vi "ASCII字符串转十六进制数组.vi"(11 "字符":string) -> (3 "数组":u8[](array[numeric]))   [LabVIEW 2015]
panel:
  out "长度":i32
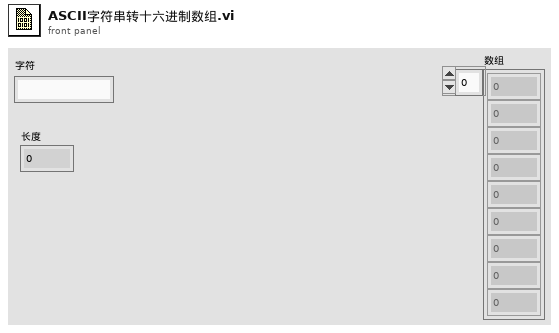
[diagram p1: front panel]
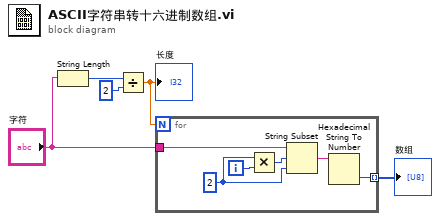
[diagram p0: block diagram]
diagram:
  n1 = String Length(string="字符") -> (length=w3:i32)
  n2 = Divide(x=w3, y=2) -> (x/y=w1:dbl)
  "长度" <- w1
  n3 = for {
    N: w1 -> [_]
    tunnel: "字符" -> [w8]
    tunnel: [w6] -> w4 mode=indexing
    i -> [w11]
    w10 = 2 ("长度（剩余）")
    n4 = Multiply(x=w10, y=w11) -> (x*y=w9:i32)
    n5 = String Subset(string=w8, offset (0)=w9, length (rest)=w10) -> (substring=w7:string)
    n6 = Hexadecimal String To Number(string=w7) -> (number=w6:u32)  [unwired: 2 in, 1 out]
  }
  "数组" <- w4
